vi "reflectionExample.vi"() -> ()   [LabVIEW 2020]
uses:
  D2/D2.lvclass
  D1/D1.lvclass
  D/D.lvclass
  C/C.lvclass
  B2/B2.lvclass
  B1/B1.lvclass
  B/B.lvclass
  A/A.lvclass
  Reflection/reflectionPool.vi
  Reflection/Reflection.lvclass
panel:
  in  "Get Hierarchy for Class:":string="D2.lvclass"
  in  "A.lvclass":refnum<class "A.lvclass">
  in  "B.lvclass":refnum<class "B.lvclass">
  in  "B1.lvclass":refnum<class "B1.lvclass">
  in  "B2.lvclass":refnum<class "B2.lvclass">
  in  "C.lvclass":refnum<class "C.lvclass">
  in  "D.lvclass":refnum<class "D.lvclass">
  in  "D1.lvclass":refnum<class "D1.lvclass">
  in  "D2.lvclass":refnum<class "D2.lvclass">
  out "classHierarchy":string[](array[string])
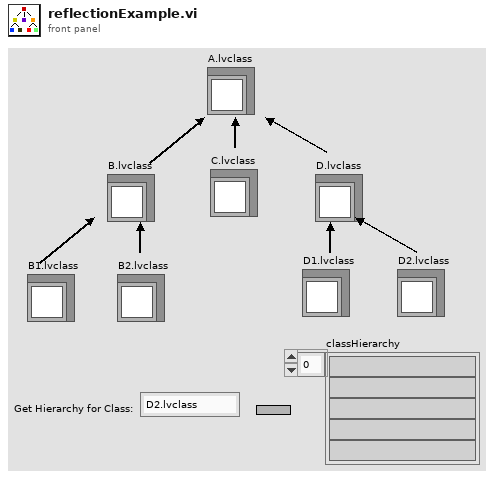
[diagram p1: front panel]
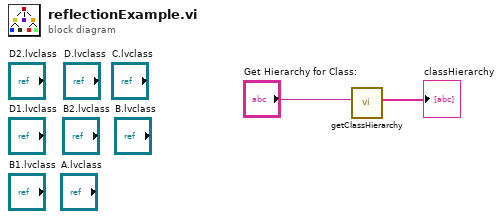
[diagram p0: block diagram]
diagram:
  n1 = call "getClassHierarchy.vi"("className"="Get Hierarchy for Class:") -> ("classHierarchy"=→"classHierarchy":string[])  [unwired: 9 in, 1 out]
